vi "Autonomous Independent.vi"() -> ()   [LabVIEW 2013]
uses:
  <vilib>/Rock Robotics/WPI/Relay/WPI_RelayValue.ctl
  <vilib>/Rock Robotics/WPI/Solenoid/WPI_SolenoidValue.ctl
  <vilib>/Rock Robotics/WPI/RobotDrive/WPI_RobotDriveGetSetRefNum.vi
  <vilib>/Rock Robotics/WPI/Solenoid/WPI_SolenoidSetEnum.vi
  <vilib>/Rock Robotics/WPI/RobotDrive/WPI_RobotDriveArcadeDrive_Standard(NoSaturation).vi
  <vilib>/Rock Robotics/WPI/DriverStation/WPI_DriverStationPositionInfo.ctl
panel:
  in  "Feet":dbl
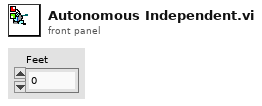
[diagram p1: front panel]
types:
  T1 = typedef "WPI_RelayValue.ctl" = enum16{"Off", "On", "Forward", "Reverse"}
  T2 = typedef "WPI_RelayDevRef.ctl" = cluster{"DevStatus":errorcluster, "Relay Channel":T3, "Digital Module":T4, "Relay Direction":T5}
  T3 = typedef "FPGA_DIORelayChannel.ctl" = enum8{"Relay 1", "Relay 2", "Relay 3", "Relay 4", "Relay 5", "Relay 6", "Relay 7", "Relay 8", "Invalid"}
  T4 = typedef "FPGA_TypedefDigitalModule.ctl" = enum16{"Digital Module 1", "Digital Module 2"}
  T5 = typedef "WPI_RelayDirection.ctl" = enum16{"Both directions", "Forward only", "Reverse only"}
  T6 = typedef "WPI_MotorControlDeviceRef.ctl" = cluster{"DeviceStatus":errorcluster, "Type":enum16{"PWM", "CAN"}, "PWM":cluster{"Digital Module":T4, "PWM Channel":T7, "DeadBand":T8}, "CAN":cluster{"Device Number":u8, "Control Mode":T9, "Semaphore":T10, "Max Vout":dbl}, "Invert":bool, "TransformRef":T11, "InvTransformRef":T11}
  T7 = typedef "FPGA_DIOPWMChannel.ctl" = enum8{"PWM 1", "PWM 2", "PWM 3", "PWM 4", "PWM 5", "PWM 6", "PWM 7", "PWM 8", "PWM 9", "PWM 10", "Invalid"}
  T8 = typedef "WPI_PWMDeadband.ctl" = cluster{"Name":string, "maxPositivePwm":i32, "minPositivePwm":i32, "centerPwm":i32, "maxNegativePwm":i32, "minNegativePwm":i32, "angularRange":u16}
  T9 = typedef "WPI_CANJaguar_ControlMode.ctl" = enum8{"Percent VBus", "Current", "Speed", "Position", "Voltage"}
  T10 = typedef "Semaphore RefNum" = refnum<k1>
  T11 = typedef "WPI_PWMTransform_ConPane.ctl" = refnum<vi>
  T12 = typedef "WPI_SolenoidDevRef.ctl" = cluster{"DevStatus":errorcluster, "Solenoid Module":T13, "Forward Solenoid Channel":T14, "Reverse Solenoid Channel":T14}
  T13 = typedef "FPGA_TypedefSolenoidModule.ctl" = enum16{"Solenoid Module 1", "Solenoid Module 2"}
  T14 = typedef "WPI_SolenoidChannel.ctl" = enum8{"Solenoid 1", "Solenoid 2", "Solenoid 3", "Solenoid 4", "Solenoid 5", "Solenoid 6", "Solenoid 7", "Solenoid 8", "Invalid"}
  T15 = typedef "WPI_DigitalInputDevRef.ctl" = cluster{"DevStatus":errorcluster, "DIO Channel":T16, "Digital Module":T4}
  T16 = typedef "FPGA_DIOChannel.ctl" = enum8{"DIO 1", "DIO 2", "DIO 3", "DIO 4", "DIO 5", "DIO 6", "DIO 7", "DIO 8", "DIO 9", "DIO 10", "DIO 11", "DIO 12", "DIO 13", "DIO 14", "Invalid"}
  T17 = typedef "WPI_RobotDriveDevRef.ctl" = cluster{"DevStatus":errorcluster, "Motors[]":T6[], "Square Inputs":bool, "Max Output":dbl, "Isochronous":bool}
  T18 = typedef "WPI_SolenoidValue.ctl" = enum16{"Off", "On", "Forward", "Reverse"}
  T19 = typedef "WPI_DriverStationPositionInfo.ctl" = enum16{"1", "2", "3"}
  T20 = typedef "WPI_AnalogChannelDevRef.ctl" = cluster{"DevStatus":errorcluster, "Analog Module":T21, "Analog Channel":T22}
  T21 = typedef "FPGA_TypedefAnalogModule.ctl" = enum16{"Analog Module 1", "Analog Module 2"}
  T22 = typedef "FPGA_AIChannel.ctl" = enum8{"AI 1", "AI 2", "AI 3", "AI 4", "AI 5", "AI 6", "AI 7", "AI 8", "Invalid"}
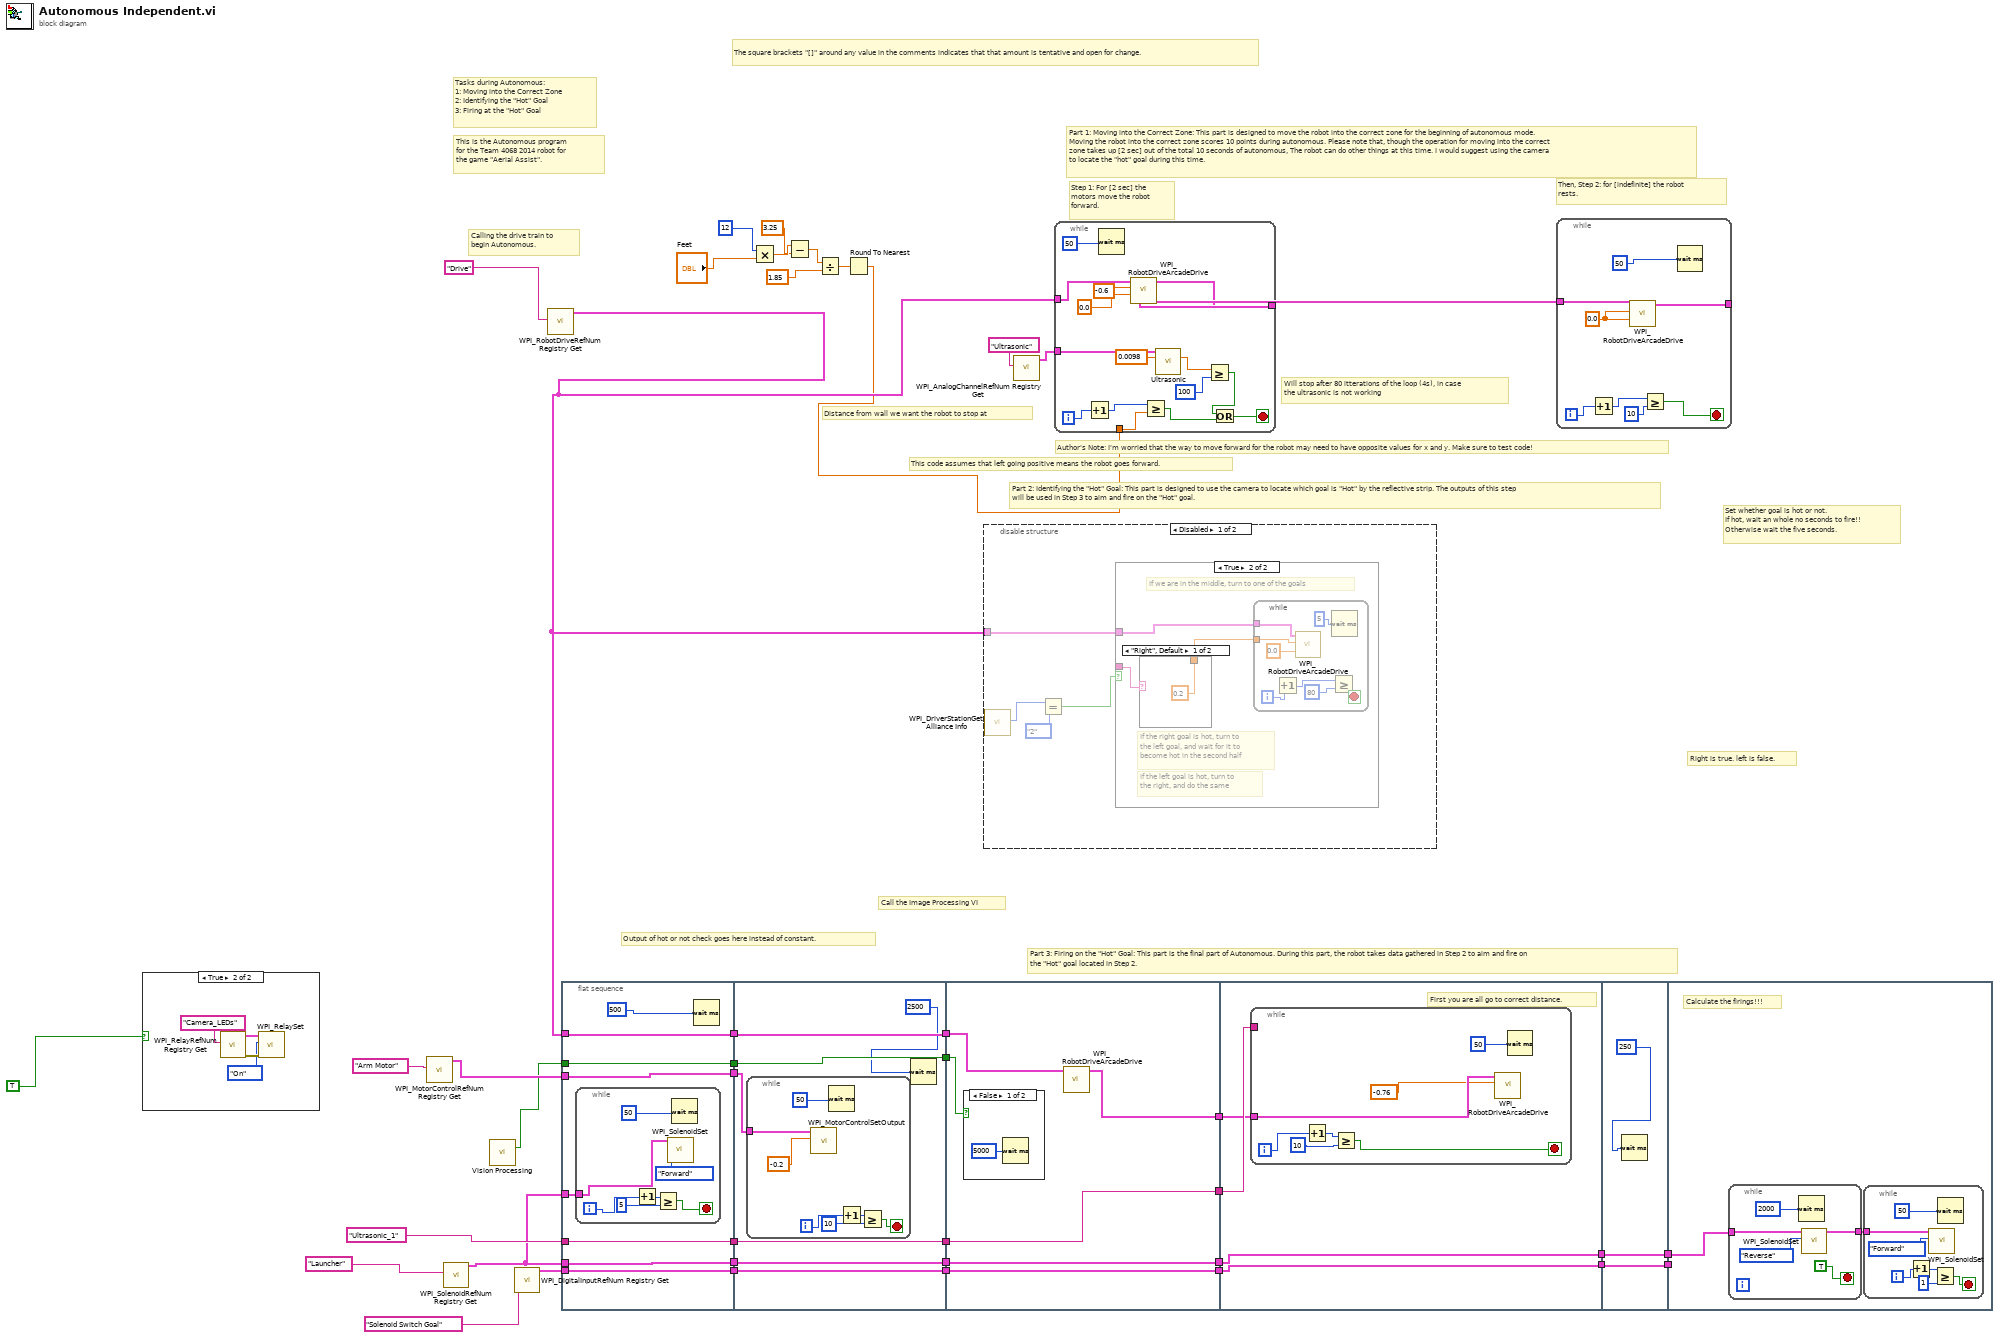
[diagram p0: block diagram]
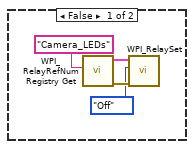
[diagram p2: hidden frame]
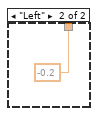
[diagram p4: hidden frame]
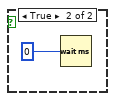
[diagram p6: hidden frame]
diagram:
  # "Will stop after 80 itterations of the loop (4s), in case\nthe ultrasonic is not working"
  # "Distance from wall we want the robot to stop at"
  # "Output of hot or not check goes here instead of constant."
  # "Call the Image Processing VI"
  # "Part 3: Firing on the \"Hot\" Goal: This part is the final part of Autonomous. During this part, the robot takes data gathered in Step 2 to aim and fire on \nthe \"Hot\" goal located in Step 2."
  # "Right is true. left is false."
  # "Set whether goal is hot or not.\nIf hot, wait an whole no seconds to fire!!\nOtherwise wait the five seconds."
  # "Part 2: Identifying the \"Hot\" Goal: This part is designed to use the camera to locate which goal is \"Hot\" by the reflective strip. The outputs of this step\nwill be used in Step 3 to aim and fire on the \"Hot\" goal."
  # "Tasks during Autonomous:\n1: Moving into the Correct Zone\n2: Identifying the \"Hot\" Goal\n3: Firing at the \"Hot\" Goal"
  # "This code assumes that left going positive means the robot goes forward."
  # "Author's Note: I'm worried that the way to move forward for the robot may need to have opposite values for x and y. Make sure to test code!"
  # "Part 1: Moving into the Correct Zone: This part is designed to move the robot into the correct zone for the beginning of autonomous mode.\nMoving the robot into the correct zone scores 10 points during autonomous. Please note that, though the operation for moving into the correct\nzone takes up [2 sec] out of the total 10 seconds of autonomous, The robot can do other things at this time. I would suggest using the camera \nto locate the \"hot\" goal during this time."
  # "The square brackets \"[]\" around any value in the comments indicates that that amount is tentative and open for change."
  # "This is the Autonomous program \nfor the Team 4068 2014 robot for \nthe game \"Aerial Assist\"."
  # "Then, Step 2: for [indefinite] the robot \nrests."
  # "Step 1: For [2 sec] the \nmotors move the robot\nforward."
  # "Calling the drive train to \nbegin Autonomous."
  n1 = case shown="True" TRUE ("LEDs") {
    frame False {
      n2 = call <vilib>:"WPI_RelayRefNum Registry Get.vi"("refnum name"="Camera_LEDs") -> ("error out"=w44:errorcluster, "RelayDevRef"=w43:T2)  [unwired: 9 in]
      n3 = call <vilib>:"WPI_RelaySet.vi"("error in (no error)"=w44, "RelayValue"=WPI_RelayValue."Off", "RelayDevRef"=w43) -> ()  [unwired: 7 in, 2 out]
    }
    frame True {
      n4 = call <vilib>:"WPI_RelayRefNum Registry Get.vi"("refnum name"="Camera_LEDs") -> ("error out"=w48:errorcluster, "RelayDevRef"=w47:T2)  [unwired: 9 in]
      n5 = call <vilib>:"WPI_RelaySet.vi"("error in (no error)"=w48, "RelayValue"=WPI_RelayValue."On", "RelayDevRef"=w47) -> ()  [unwired: 7 in, 2 out]
    }
  }
  n6 = call <vilib>:"WPI_MotorControlRefNum Registry Get.vi"("refnum name"="Arm Motor") -> ("MotorControlDevRef"=w17:T6)  [unwired: 9 in, 1 out]
  n7 = call <vilib>:"WPI_SolenoidRefNum Registry Get.vi"("refnum name"="Launcher") -> ("SolenoidDevRef"=w14:T12)  [unwired: 9 in, 1 out]
  n8 = call "Vision Processing.vi"() -> ("goal hot"=w2:bool)  [unwired: 26 in, 1 out]
  n9 = call <vilib>:"WPI_DigitalInputRefNum Registry Get.vi"("refnum name"="Solenoid Switch Goal") -> ("DigitalInputDevRef"=w19:T15)  [unwired: 9 in, 1 out]
  n10 = call <vilib>:"WPI_RobotDriveRefNum Registry Get.vi"("refnum name"="Drive") -> ("RobotDriveDevRef"=w11:T17)  [unwired: 9 in, 1 out]
  n11 = flat-sequence {
    tunnel: w17 -> [w53]
    tunnel: w19 -> [w54]
    tunnel: w2 -> [w55]
    tunnel: "Ultrasonic_1" -> [w56]
    tunnel: w11 -> [w57]
    tunnel: [w57] -> w39
    tunnel: [w56] -> w38
    tunnel: [w55] -> w37
    tunnel: [w54] -> w36
    tunnel: [w53] -> w35
    tunnel: w14 -> [w51]
    tunnel: [w50] -> w34
    tunnel: w14 -> [w50]
    tunnel: [w71] -> w33
    tunnel: [w70] -> w32
    tunnel: [w69] -> w31
    tunnel: [w68] -> w30
    tunnel: w39 -> [w71]
    tunnel: w38 -> [w70]
    tunnel: w37 -> [w69]
    tunnel: w36 -> [w68]
    tunnel: w35 -> [w66]
    tunnel: w34 -> [w65]
    tunnel: [w65] -> w29
    tunnel: [w83] -> w28
    tunnel: [w81] -> w27
    tunnel: [w80] -> w26
    tunnel: w33 -> [w84]
    tunnel: w32 -> [w83]
    tunnel: w31 -> [w82]
    tunnel: w30 -> [w80]
    tunnel: [w79] -> w25
    tunnel: w29 -> [w79]
    tunnel: w28 -> [w90]
    tunnel: w27 -> [w89]
    tunnel: w26 -> [w88]
    tunnel: [w88] -> w24
    tunnel: w25 -> [w87]
    tunnel: [w87] -> w23
    tunnel: [w99] -> w22
    tunnel: w24 -> [w99]
    tunnel: [w98] -> w21
    tunnel: w23 -> [w98]
    tunnel: w22 -> [_]
    tunnel: w21 -> [w101]
    frame #0 {
      n12 = while {
        tunnel: w51 -> [w59]
        i -> [w61]
        stop <- w60 stop-if-true
        n13 = Increment(x=w61) -> (x+1=w63:i32)
        n14 = Greater Or Equal?(x=w63, y=5) -> (x >= y?=w60:bool)
        n15 = call-poly <vilib>:"WPI_SolenoidSet.vi"("Value"=WPI_SolenoidValue."Forward", "SolenoidDevRef"=w59) -> ()  [unwired: 8 in, 2 out]
        n16 = Wait (ms)(milliseconds to wait=50) -> ()  [unwired: 1 out]
      }
      n17 = Wait (ms)(milliseconds to wait=500) -> ()  [unwired: 1 out]
    }
    frame #1 {
      n18 = while {
        tunnel: w66 -> [w73]
        i -> [w78]
        stop <- w75 stop-if-true
        n19 = call <vilib>:"WPI_MotorControlSetOutput.vi"("Output"=-0.2, "MotorControlDevRef"=w73) -> ()  [unwired: 7 in, 3 out]
        n20 = Wait (ms)(milliseconds to wait=50) -> ()  [unwired: 1 out]
        n21 = Increment(x=w78) -> (x+1=w77:i32)
        n22 = Greater Or Equal?(x=w77, y=10) -> (x >= y?=w75:bool)
      }
      n23 = Wait (ms)(milliseconds to wait=2500) -> ()  [unwired: 1 out]
    }
    frame #2 {
      n24 = case shown="False" w82 {
        frame False {
          n25 = Wait (ms)(milliseconds to wait=5000) -> ()  [unwired: 1 out]
        }
        frame True {
          n26 = Wait (ms)(milliseconds to wait=0) -> ()  [unwired: 1 out]
        }
      }
      n27 = call-poly <vilib>:"WPI_RobotDriveArcadeDrive.vi"("RobotDriveDevRef"=w84) -> ("RobotDriveDevRef"=w81:T17)  [unwired: 8 in, 2 out]
    }
    frame #3 {
      # "First you are all go to correct distance."
      n28 = while {
        tunnel: w90 -> [_]
        tunnel: w89 -> [w97]
        i -> [w94]
        stop <- w91 stop-if-true
        n29 = Increment(x=w94) -> (x+1=w93:i32)
        n30 = Greater Or Equal?(x=w93, y=10) -> (x >= y?=w91:bool)
        n31 = call-poly <vilib>:"WPI_RobotDriveArcadeDrive.vi"("X axis value"=-0.76, "RobotDriveDevRef"=w97) -> ()  [unwired: 7 in, 3 out]
        n32 = Wait (ms)(milliseconds to wait=50) -> ()  [unwired: 1 out]
      }
    }
    frame #4 {
      n33 = Wait (ms)(milliseconds to wait=250) -> ()  [unwired: 1 out]
    }
    frame #5 {
      # "Calculate the firings!!!"
      n34 = while {
        tunnel: w101 -> [w114]
        tunnel: [w113] -> w102
        stop <- TRUE stop-if-true
        n35 = Wait (ms)(milliseconds to wait=2000) -> ()  [unwired: 1 out]
        n36 = call-poly <vilib>:"WPI_SolenoidSet.vi"("Value"=WPI_SolenoidValue."Reverse", "SolenoidDevRef"=w114) -> ("SolenoidDevRef"=w113:T12)  [unwired: 8 in, 1 out]
      }
      n37 = while {
        tunnel: w102 -> [w109]
        i -> [w107]
        stop <- w104 stop-if-true
        n38 = Increment(x=w107) -> (x+1=w106:i32)
        n39 = call-poly <vilib>:"WPI_SolenoidSet.vi"("Value"=WPI_SolenoidValue."Forward", "SolenoidDevRef"=w109) -> ()  [unwired: 8 in, 2 out]
        n40 = Greater Or Equal?(x=w106, y=1) -> (x >= y?=w104:bool)
        n41 = Wait (ms)(milliseconds to wait=50) -> ()  [unwired: 1 out]
      }
    }
  }
  n42 = Multiply(x=12, y="Feet") -> (x*y=w7:dbl)
  n43 = Subtract(x=w7, y=3.25) -> (x-y=w5:dbl)
  n44 = Divide(x=w5, y=1.85) -> (x/y=w4:dbl)
  n45 = Round To Nearest(number=w4) -> (nearest integer value=w3:dbl)
  n46 = disable-structure shown="Disabled" {
    disable-tunnel: w11 -> [w115 _]
    frame Disabled {
      n47 = call <vilib>:"WPI_DriverStationGet Alliance Info.vi"() -> ("Position"=w118:T19)  [unwired: 10 in, 1 out]
      n48 = Equal?(x=w118, y=WPI_DriverStationPositionInfo."2") -> (x = y?=w116:bool)
      n49 = case shown="True" w116 {
        tunnel: w115 -> [_ w121]
        tunnel: _ -> [_ w120]
        frame False {
        }
        frame True {
          # "If the left goal is hot, turn to\nthe right, and do the same"
          # "If the right goal is hot, turn to\nthe left goal, and wait for it to\nbecome hot in the second half"
          # "If we are in the middle, turn to one of the goals"
          n50 = case shown="\"Right\", Default" w120 {
            tunnel: [0.2 -0.2] -> w119
            frame "Right", Default {
            }
            frame "Left" {
            }
          }
          n51 = while {
            tunnel: w121 -> [w131]
            tunnel: w119 -> [w124]
            i -> [w127]
            stop <- w126 stop-if-true
            n52 = Increment(x=w127) -> (x+1=w129:i32)
            n53 = call-poly <vilib>:"WPI_RobotDriveArcadeDrive.vi"("Y axis value"=0.0, "X axis value"=w124, "RobotDriveDevRef"=w131) -> ()  [unwired: 6 in, 3 out]
            n54 = Greater Or Equal?(x=w129, y=80) -> (x >= y?=w126:bool)
            n55 = Wait (ms)(milliseconds to wait=u32 5) -> ()  [unwired: 1 out]
          }
        }
      }
    }
    frame Enabled {
    }
  }
  n56 = call <vilib>:"WPI_AnalogChannelRefNum Registry Get.vi"("refnum name"="Ultrasonic") -> ("AIDeviceRef"=w12:T20)  [unwired: 9 in, 1 out]
  n57 = while {
    tunnel: w11 -> [w146]
    tunnel: [w145] -> w40
    tunnel: w12 -> [w139]
    tunnel: w3 -> [w132]
    i -> [w144]
    stop <- w137 stop-if-true
    n58 = Increment(x=w144) -> (x+1=w143:i32)
    n59 = Wait (ms)(milliseconds to wait=50) -> ()  [unwired: 1 out]
    n60 = call-poly <vilib>:"WPI_RobotDriveArcadeDrive.vi"("Y axis value"=0.0, "X axis value"=-0.6, "RobotDriveDevRef"=w146) -> ("RobotDriveDevRef"=w145:T17)  [unwired: 6 in, 2 out]
    n61 = Greater Or Equal?(x=w143, y=w132) -> (x >= y?=w138:bool)
    n62 = call "Ultrasonic.vi"("AIDeviceRef"=w139, "Scaling factor (Vcc/cm)"=0.0098 ("Scaling factor (V/in)")) -> ("Distance"=w134:dbl)  [unwired: 11 in, 2 out]
    n63 = Greater Or Equal?(x=w134, y=100) -> (x >= y?=w136:bool)
    n64 = Or(x=w136, y=w138) -> (x .or. y?=w137:bool)
  }
  n65 = while {
    tunnel: w40 -> [w154]
    tunnel: [w152] -> _
    i -> [w150]
    stop <- w147 stop-if-true
    w153 = 0.0
    n66 = Increment(x=w150) -> (x+1=w148:i32)
    n67 = call-poly <vilib>:"WPI_RobotDriveArcadeDrive.vi"("Y axis value"=w153, "X axis value"=w153, "RobotDriveDevRef"=w154) -> ("RobotDriveDevRef"=w152:T17)  [unwired: 6 in, 2 out]
    n68 = Greater Or Equal?(x=w148, y=10) -> (x >= y?=w147:bool)
    n69 = Wait (ms)(milliseconds to wait=50) -> ()  [unwired: 1 out]
  }
